vi "TDT-Connect ZBUS.vi"(11 "error in (no error)":errorcluster) -> (8 "ZBUSx":refnum<k7>, 15 "error out":errorcluster)   [LabVIEW 2020]
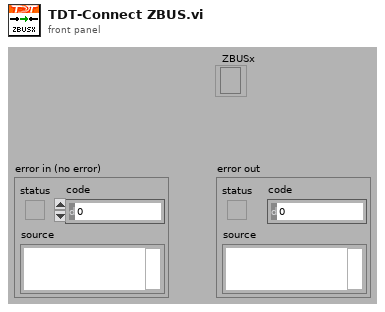
[diagram p1: front panel]
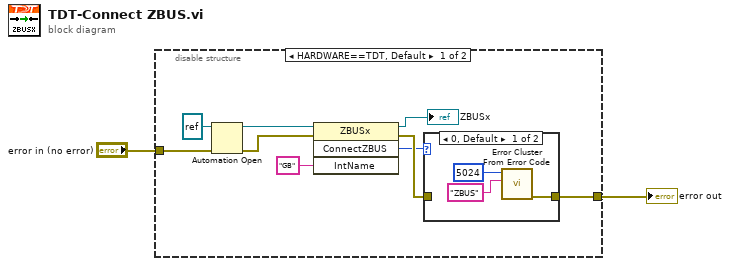
[diagram p0: block diagram]
diagram:
  n1 = disable-structure shown="HARDWARE==TDT, Default" {
    disable-tunnel: "error in (no error)" -> [w11 w16]
    disable-tunnel: [w3 w16] -> w1
    frame condition #0 (active) {
      n2 = Automation Open(error in (no error)=w11, Automation Refnum=refnum<k7> refnum ("ZBUSXLib.ZBUSx")) -> (Automation Refnum=w5:refnum<k7>, error out=w7:errorcluster)  [unwired: 2 in]
      n3 = invoke class="ZBUSx" method="ConnectZBUS"(reference=w5, error in=w7, "IntName"="GB" ("ServerName")) -> (reference out=→"ZBUSx":refnum<k7>, error out=w9:errorcluster, "ConnectZBUS"=w8:i32)  [unwired: 1 in, 1 out]
      n4 = case shown="0, Default" w8 {
        tunnel: w9 -> [_ w15]
        tunnel: [w12 w15] -> w3
        frame 0, Default {
          n5 = call <vilib>:"Error Cluster From Error Code.vi"("error message (\"\")"="ZBUS" ("error message (\"\")"), "error code (0)"=5024) -> ("error out"=w12:errorcluster)  [unwired: 7 in]
        }
        frame 1 {
        }
      }
    }
    frame condition #1 {
    }
  }
  "error out" <- w1
